vi "Is Actor.vi"(8 "error in (no error)":errorcluster, 9 "Validation":T1, 11 "ProjectItem in":refnum<vi>) -> (0 "error out":errorcluster, 1 "Has Public Methods":bool, 2 "Is Actor":bool, 3 "ProjectItem out":refnum<vi>, 4 "Is Actor Interface":bool)   [LabVIEW 2020, in "Actor Message Maker Provider.lvlib"]
uses:
  Actor Message Maker Provider.lvlib
  MessageMakerProvider/_Message Maker/Message Maker.lvlib
  MessageMakerProvider/AFPP Shared/Validation Mode.ctl
  MessageMakerProvider/AFPP Shared/AFPP Shared.lvlib
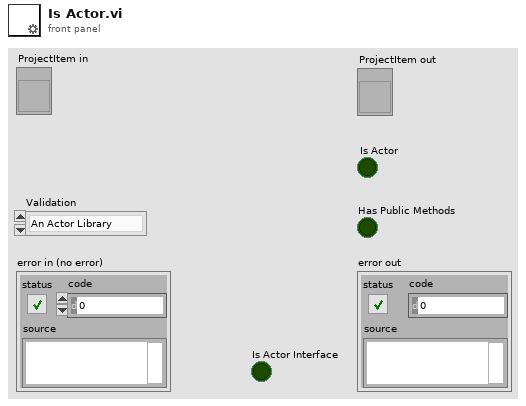
[diagram p1: front panel]
types:
  T1 = typedef "AFPP Shared.lvlib/Validation Mode.ctl" = enum16{"An Actor Library", "A Target Tag"}
  T2 = enum32{"invalid scope", "public", "private", "protected", "community"}
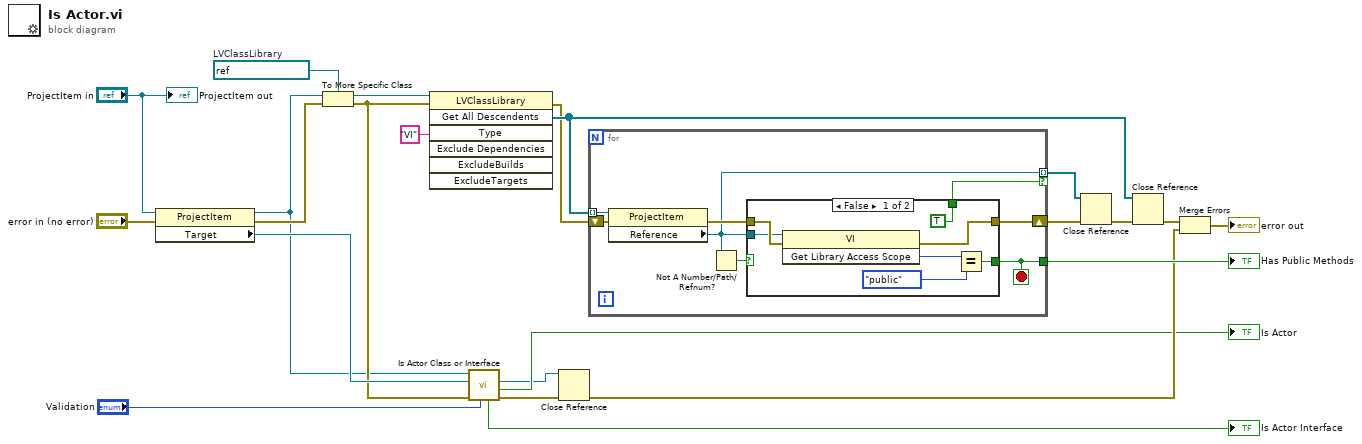
[diagram p0: block diagram]
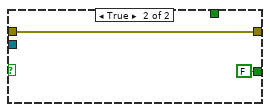
[diagram p2: hidden frame]
diagram:
  w23 = refnum<vi> refnum  # LVClassLibrary
  n1 = property class="ProjectItem"(reference="ProjectItem in", error in="error in (no error)") -> (reference out=w8:refnum<vi>, error out=w14:errorcluster, "Target"=w16:refnum<vi>)
  n2 = To More Specific Class(target class=w23, reference=w8, error in=w14) -> (specific class reference=w18:refnum<vi>, error out=w13:errorcluster)
  n3 = invoke class="LVClassLibrary" method="Get All Descendents"(reference=w18, error in=w13, "Type"="VI") -> (error out=w19:errorcluster, "All Descendents"=w20:refnum<vi>[])  [unwired: 4 in, 5 out]
  n4 = call "Is Actor Class or Interface.vi"("Validation"="Validation", "error in (no error)"=w13, "Target in"=w16, "LVClass Library in"=w8) -> ("error out"=w15:errorcluster, "is actor?"=→"Is Actor":bool, "TargetItem out"=w5:refnum<vi>, "is actor interface?"=→"Is Actor Interface":bool)  [unwired: 4 in]
  n5 = Close Reference(reference=w5, error in (no error)=w15) -> (error out=w11:errorcluster)
  n6 = for {
    tunnel: [w29] -> w22
    tunnel: w20 -> [w27] mode=indexing
    shift-right: [w26] -> w3
    shift-left: w19 -> [w28]
    tunnel: [w25] -> w1 mode=indexing if=w24
    stop <- w29 stop-if-true
    n7 = property class="ProjectItem"(reference=w27, error in=w28) -> (error out=w31:errorcluster, "Reference"=w25:refnum<vi>)  [unwired: 1 out]
    n8 = Not A Number/Path/Refnum?(number/path/refnum=w25) -> (NaN/Path/Refnum?=w30:bool)
    n9 = case shown="False" w30 {
      tunnel: w25 -> [w33 _]
      tunnel: w31 -> [w38 w40]
      tunnel: [w34 w40] -> w26
      tunnel: [w35 FALSE] -> w29
      tunnel: [TRUE _] -> w24
      frame False {
        n10 = invoke class="VI" method="Get Library Access Scope"(reference=w33, error in=w38) -> (error out=w34:errorcluster, "Get Library Access Scope"=w37:T2)  [unwired: 1 in, 1 out]
        n11 = Equal?(x=w37, y=T2."public") -> (x = y?=w35:bool)
      }
      frame True {
      }
    }
  }
  "Has Public Methods" <- w22
  n12 = Close Reference(reference=w1, error in (no error)=w3) -> (error out=w2:errorcluster)
  n13 = Close Reference(reference=w20, error in (no error)=w2) -> (error out=w12:errorcluster)
  n14 = Merge Errors(w12, w11) -> (→"error out":errorcluster)
  "ProjectItem out" <- "ProjectItem in"
